vi "GetLabels.vi"(0 "Array":T1(array[cluster]), 1 "Region of Interest":i32) -> (2 "Region Labels":string[](array[string]), 3 "No. of regions":i32, 4 "Strip Labels":string[](array[string]), 5 "No. of Points":i32)   [LabVIEW 2019]
doc: "Utility to read the labels of probe regions and strips."
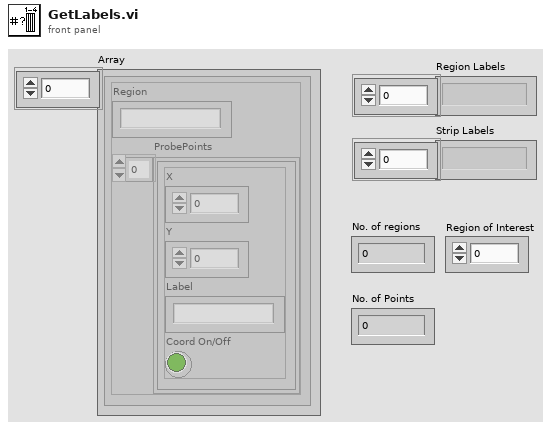
[diagram p1: front panel]
types:
  T1 = cluster{"Region":string, "ProbePoints":cluster{"X":dbl, "Y":dbl, "Label":string, "Coord On/Off":bool}[]}[]
  T2 = cluster{"X":dbl, "Y":dbl, "Label":string, "Coord On/Off":bool}[]
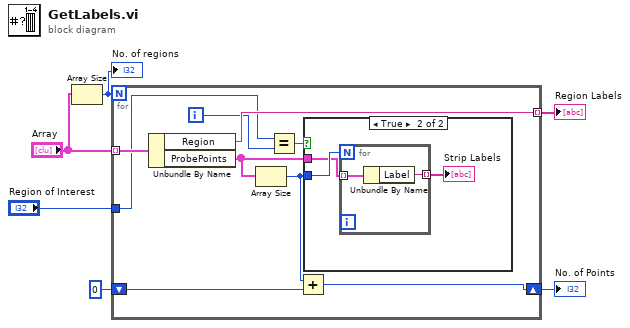
[diagram p0: block diagram]
diagram:
  n1 = Array Size(array="Array") -> (size(s)=w4:i32)
  "No. of regions" <- w4
  n2 = for {
    N: w4 -> [_]
    tunnel: "Array" -> [w15] mode=indexing
    tunnel: [w14] -> w5 mode=indexing
    shift-right: [w13] -> w2
    shift-left: 0 -> [w12]
    tunnel: "Region of Interest" -> [w8]
    i -> [w7]
    n3 = Unbundle By Name(w15) -> ("Region"=w14:string, "ProbePoints"=w10:T2)
    n4 = Array Size(array=w10) -> (size(s)=w11:i32)
    n5 = Equal?(x=w8, y=w7) -> (x = y?=w9:bool)
    n6 = Add(x=w11, y=w12) -> (x+y=w13:i32)
    n7 = case shown="True" w9 {
      tunnel: w11 -> [_ w18]
      tunnel: w10 -> [_ w17]
      frame False {
      }
      frame True {
        n8 = for {
          N: w18 -> [_]
          tunnel: w17 -> [w20] mode=indexing
          tunnel: [w19] -> w16 mode=indexing
          n9 = Unbundle By Name(w20) -> ("Label"=w19:string)
        }
        "Strip Labels" <- w16
      }
    }
  }
  "Region Labels" <- w5
  "No. of Points" <- w2
